vi "Sequence Execution Example.vi"() -> ()   [LabVIEW 2010]
panel:
  out "3":bool
  out "4":bool
  out "2":bool
  out "1":bool
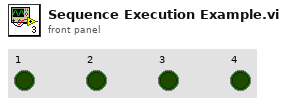
[diagram p1: front panel]
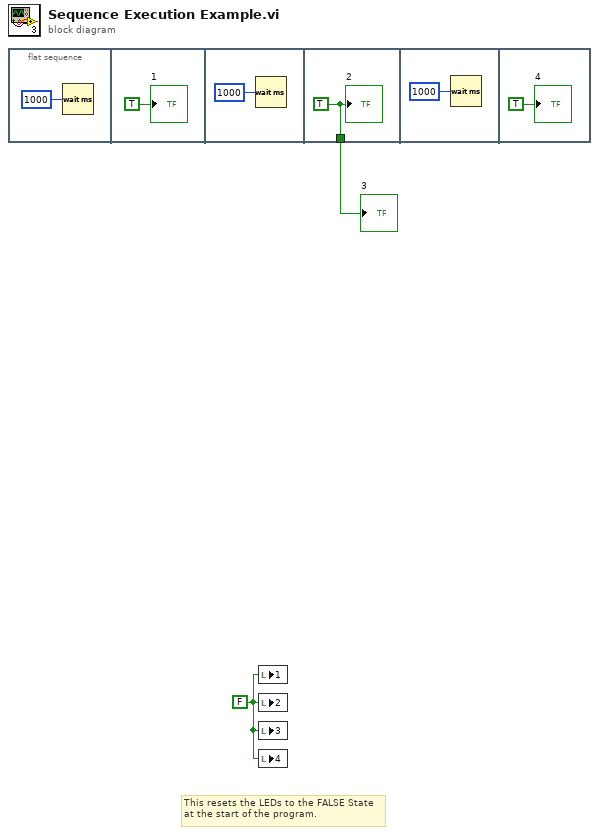
[diagram p0: block diagram]
diagram:
  w1 = FALSE
  # "This resets the LEDs to the FALSE State\nat the start of the program."
  n1 = flat-sequence {
    tunnel: [w6] -> w2
    frame #0 {
      n2 = Wait (ms)(milliseconds to wait=u32 1000) -> ()  [unwired: 1 out]
    }
    frame #1 {
      "1" <- TRUE
    }
    frame #2 {
      n3 = Wait (ms)(milliseconds to wait=u32 1000) -> ()  [unwired: 1 out]
    }
    frame #3 {
      w6 = TRUE
      "2" <- w6
    }
    frame #4 {
      n4 = Wait (ms)(milliseconds to wait=u32 1000) -> ()  [unwired: 1 out]
    }
    frame #5 {
      "4" <- TRUE
    }
  }
  n5 = local write "1"(w1) -> ()
  n6 = local write "2"(w1) -> ()
  n7 = local write "3"(w1) -> ()
  n8 = local write "4"(w1) -> ()
  "3" <- w2
